vi "Create Host Stream Command Queue.vi"(8 "error in (no error)":errorcluster) -> (0 "error out":errorcluster, 3 "Cmd Q":refnum<queue>)   [LabVIEW 2019, in "CAN Streaming Support Workspace Shared.lvlib"]
uses:
  CAN Streaming Support Workspace Shared.lvlib
  Types/Host Stream API Queue Cmd.ctl
  Types/Host Stream API Queue Type.ctl
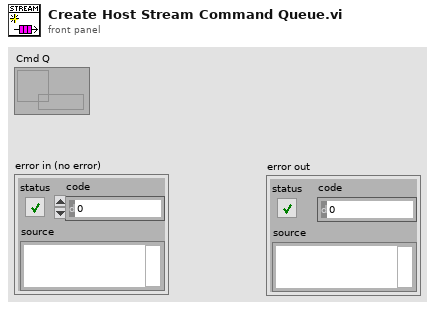
[diagram p1: front panel]
types:
  T1 = typedef "CAN Streaming Support Workspace Shared.lvlib/Host Stream API Queue Type.ctl" = cluster{"Cmd":T2, "Target IP Address":string, "Addon":string}
  T2 = typedef "CAN Streaming Support Workspace Shared.lvlib/Host Stream API Queue Cmd.ctl" = enum8{"Start Stream", "Stop Stream", "Exit"}
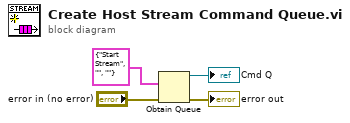
[diagram p0: block diagram]
diagram:
  n1 = Obtain Queue(element data type=T1 {"Cmd"=enum."Start Stream", "Target IP Address"="", "Addon"=""}, error in (no error)="error in (no error)") -> (queue out=→"Cmd Q":refnum<queue>, error out=→"error out":errorcluster)  [unwired: 3 in, 1 out]
